vi "Create Notifier.vi"(8 "error in (no error)":errorcluster) -> (0 "error out":errorcluster, 3 "notifier out":refnum<notifier>)   [LabVIEW 2021]
doc: "Create a boolean user event that will be used to stop the event loop from the message handling loop."
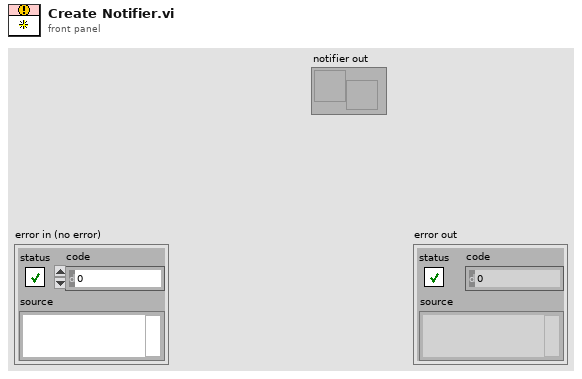
[diagram p1: front panel]
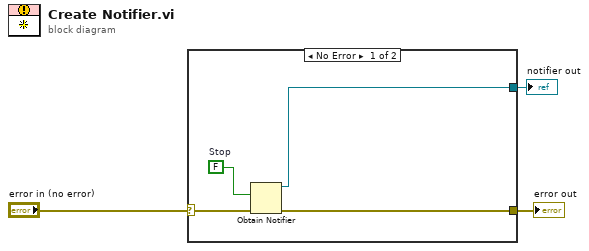
[diagram p0: block diagram]
diagram:
  n1 = case shown="No Error" "error in (no error)" {
    selector: "error in (no error)" -> [w5 w8]
    tunnel: [w7 _] -> w1
    tunnel: [w6 w8] -> w3
    frame No Error {
      w4 = FALSE  # Stop
      n2 = Obtain Notifier(notification data type=w4, error in (no error)=w5) -> (notifier out=w7:refnum<notifier>, error out=w6:errorcluster)  [unwired: 2 in, 1 out]
    }
    frame Error {
    }
  }
  "error out" <- w3
  "notifier out" <- w1
